vi "pause4.vi"() -> ()   [LabVIEW 2020]
panel:
  in  "pause4":bool
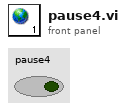
[diagram p1: front panel]
diagram:
